vi "Teleop.vi"(10 "Match Info":T1={"Autonomous Elapsed Seconds"=0.0, "TeleOp Elapsed Seconds"=0.0, "Disabled Elapsed Seconds"=0.0, "Visited Autonomous"=FALSE, "Visited TeleOp"=FALSE, "Visited Disabled"=FALSE, "Autonomous Settings"={"Autonomous Style"=enum."Independent", "VI Refnum"=refnum}}, 11 "Call Context":T2) -> ()   [LabVIEW 2019]
doc: "This VI is called for each TeleOp packet received from the DS where the robot is not disabled. It is often used to read from the joysticks and update I/O or to update setpoints for timed control loops. It should complete and return within 20 milliseconds or it may miss DS packets."
uses:
  <vilib>/Rock Robotics/WPI/DriverStation/WPI_DriverStationDerivedRobotMode.ctl
  <vilib>/Rock Robotics/WPI/DriverStation/WPI_DriverStationMatch Info.ctl
  Robot Global Data.vi
  <vilib>/Rock Robotics/Network Tables/NT Write Number.vi
  <vilib>/Rock Robotics/WPI/Utilities/WPI_GetSetVariantRefNum.vi
panel:
  in  "Chassis X SPD":dbl=0.65
  in  "Chassis Y SPD":dbl=0.7
  # "Click here to set max"
  # "Click here to set min"
  # "Click here to set max"
  # "Click here to set min"
  # "Click here to set max"
  # "Click here to set min"
  # "Click here to set max"
  # "Click here to set min"
  # "Click here to set max"
  # "Click here to set min"
  # "Click here to set max"
  # "Click here to set min"
  # "Click here to set max"
  # "Click here to set min"
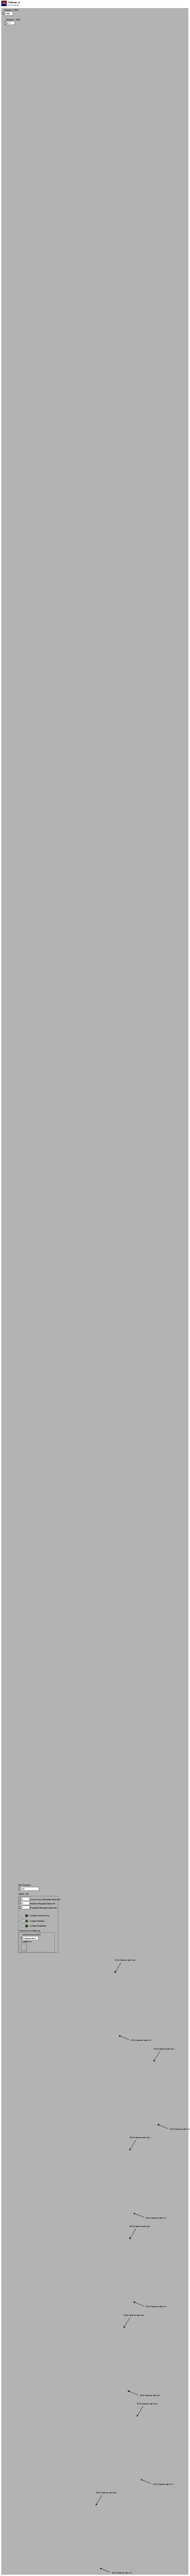
[diagram p1: front panel]
types:
  T1 = typedef "WPI_DriverStationMatch Info.ctl" = cluster{"Autonomous Elapsed Seconds":dbl, "TeleOp Elapsed Seconds":dbl, "Disabled Elapsed Seconds":dbl, "Visited Autonomous":bool, "Visited TeleOp":bool, "Visited Disabled":bool, "Autonomous Settings":cluster{"Autonomous Style":enum16{"Iterative", "Independent"}, "VI Refnum":refnum<vi>}}
  T2 = typedef "WPI_DriverStationDerivedRobotMode.ctl" = enum16{"Init", "Execute", "Stop"}
  T3 = typedef "WPI_MotorControlDeviceRef.ctl" = cluster{"DeviceStatus":errorcluster, "Type":T4, "PWM":cluster{"PWM Channel":T5, "DeadBand":T6}, "CAN":cluster{"Device Number":u8, "SetOutput VI Ref":variant, "GetOutput VI Ref":variant, "Enable VI Ref":variant, "Disable VI Ref":variant, "Data":variant}, "Invert":bool, "DIO PWM":cluster{"PWM \"Enable\" Channel":T5, "DIOChannel":T7, "PWM Rate":dbl}}
  T4 = typedef "WPI_MotorControlType.ctl" = enum16{"PWM", "CAN", "DIO PWM"}
  T5 = typedef "FPGA_DIOPWMChannel.ctl" = enum8{"PWM 0", "PWM 1", "PWM 2", "PWM 3", "PWM 4", "PWM 5", "PWM 6", "PWM 7", "PWM 8", "PWM 9", "PWM MXP 0", "PWM MXP 1", "PWM MXP 2", "PWM MXP 3", "PWM MXP 4", "PWM MXP 5", "PWM MXP 6", "PWM MXP 7", "PWM MXP 8", "PWM MXP 9", "Invalid"}
  T6 = typedef "WPI_PWMDeadband.ctl" = cluster{"Name":string, "maxPositivePwm":i32, "minPositivePwm":i32, "centerPwm":i32, "maxNegativePwm":i32, "minNegativePwm":i32, "angularRange":u16}
  T7 = typedef "FPGA_DIOChannel.ctl" = enum8{"DIO 0", "DIO 1", "DIO 2", "DIO 3", "DIO 4", "DIO 5", "DIO 6", "DIO 7", "DIO 8", "DIO 9", "DIO MXP 0", "DIO MXP 1", "DIO MXP 2", "DIO MXP 3", "DIO MXP 4", "DIO MXP 5", "DIO MXP 6", "DIO MXP 7", "DIO MXP 8", "DIO MXP 9", "DIO MXP 10", "DIO MXP 11", "DIO MXP 12", "DIO MXP 13", "DIO MXP 14", "DIO MXP 15", "SPI Port CS1", "SPI Port CS2", "SPI Port CS3", "SPI Port MISO", "SPI Port MOSI", "Invalid"}
  T8 = typedef "WPI_ServoDeviceRef.ctl" = cluster{"DeviceStatus":errorcluster, "PWM Channel":T5, "DeadBand":T6}
  T9 = typedef "WPI_JoystickDevRef.ctl" = cluster{"Device":T10}
  T10 = typedef "WPI_JoystickDeviceEnum.ctl" = enum16{"USB 0", "USB 1", "USB 2", "USB 3", "USB 4", "USB 5"}
  T11 = typedef "WPI_RobotDriveDevRef.ctl" = cluster{"DevStatus":errorcluster, "Motors[]":T3[], "Square Inputs":bool, "Max Output":dbl}
  T12 = cluster{"JoystickDevRef":T9, "RobotDriveDevRef":T11}
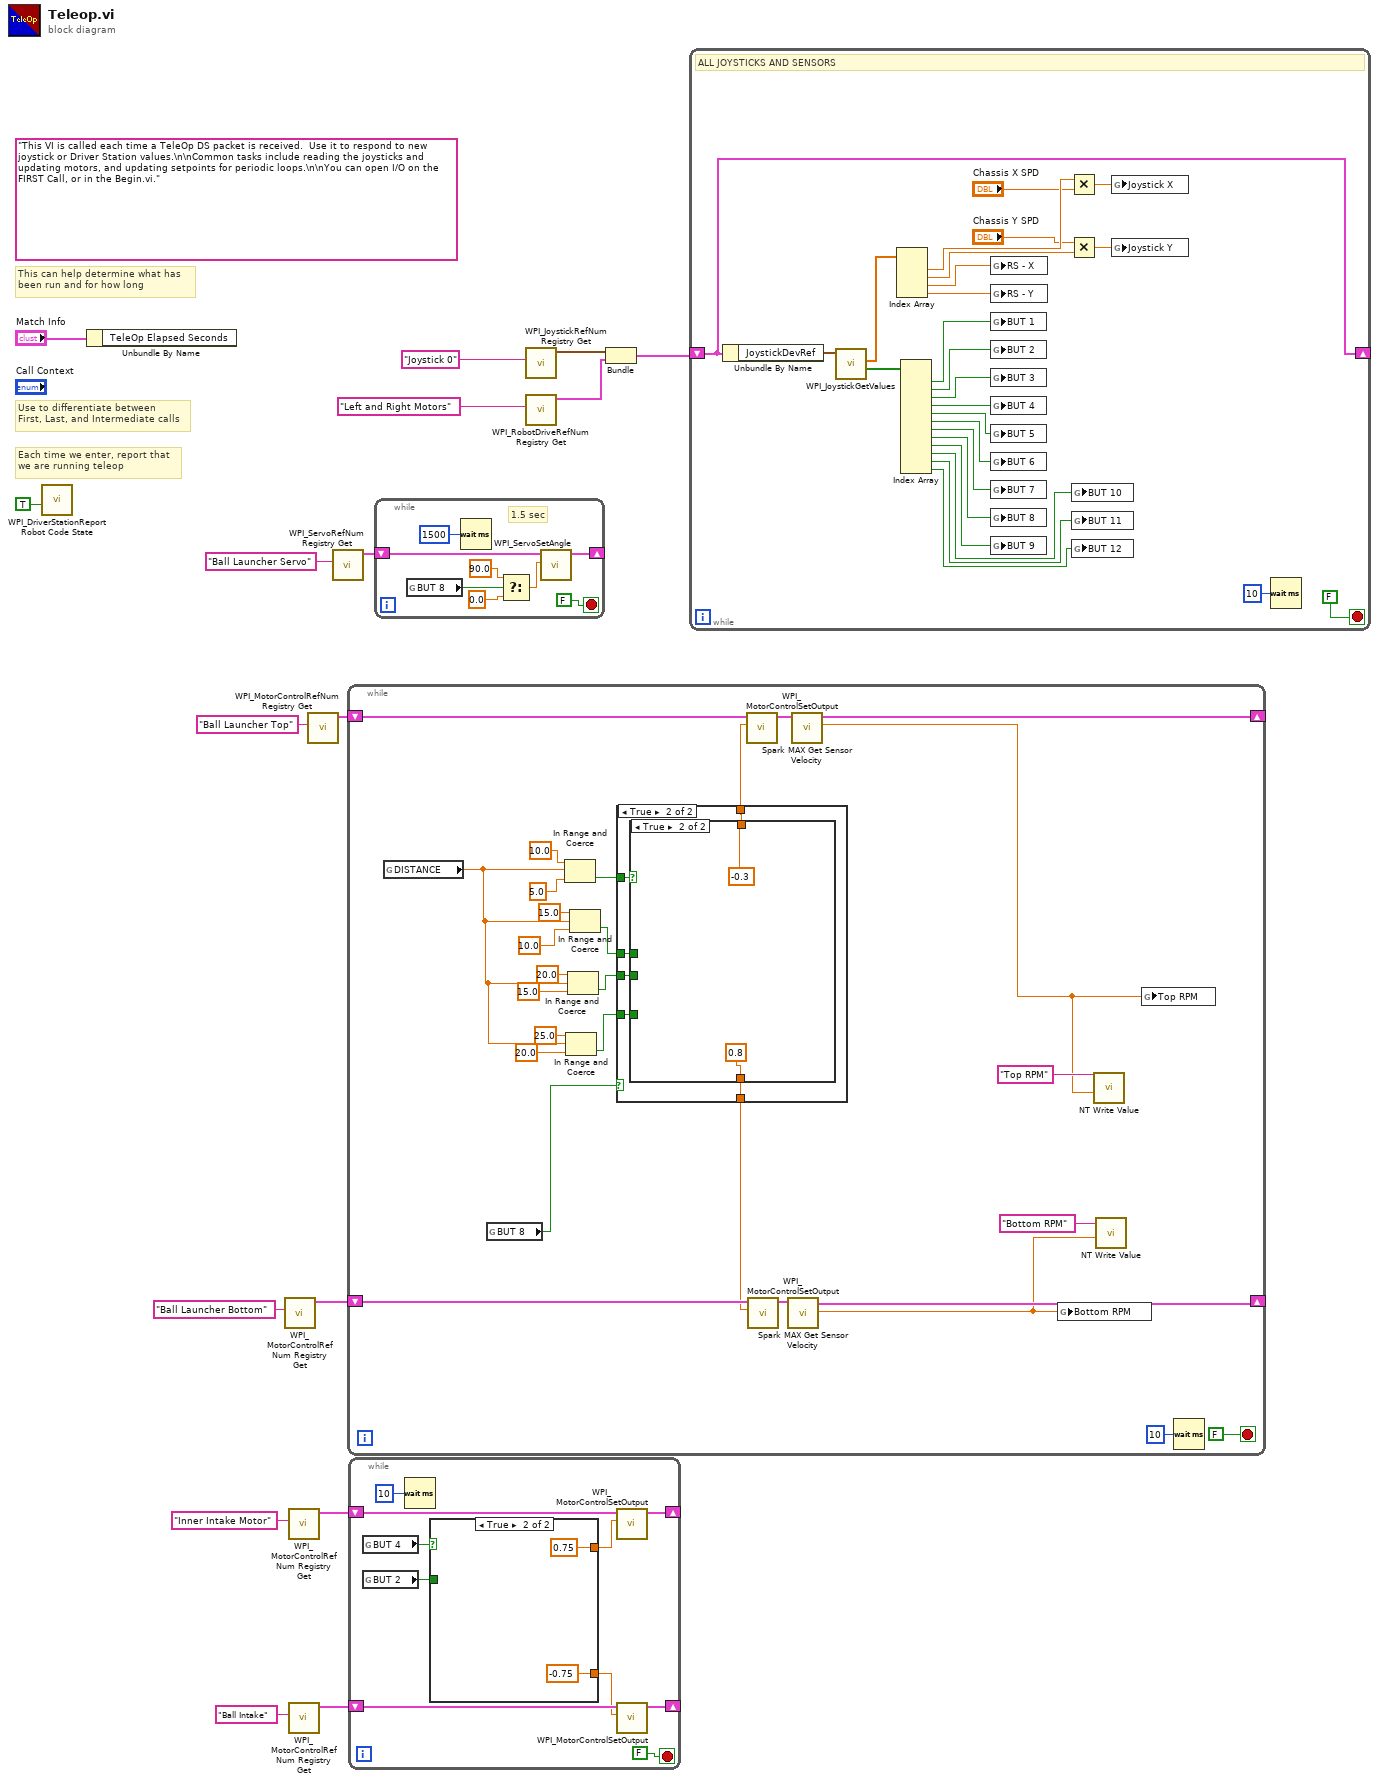
[diagram p0: block diagram]
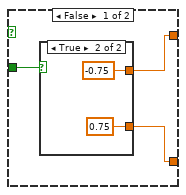
[diagram p2: hidden frame]
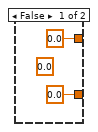
[diagram p3: hidden frame]
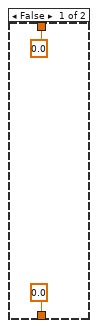
[diagram p4: hidden frame]
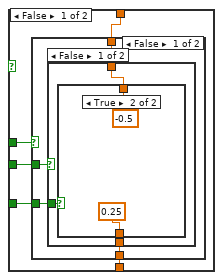
[diagram p5: hidden frame]
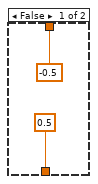
[diagram p6: hidden frame]
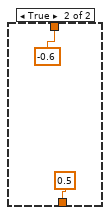
[diagram p7: hidden frame]
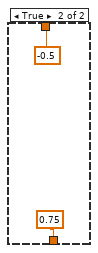
[diagram p8: hidden frame]
diagram:
  (unwired) "This VI is called each time a TeleOp DS packet is received.  Use it to respond to new joystick or Driver Station values.\n\nCommon tasks include reading the joysticks and updating motors, and updating setpoints for periodic loops.\n\nYou can open I/O on the FIRST Call, or in the Begin.vi."
  # "Each time we enter, report that\nwe are running teleop"
  # "Use to differentiate between\nFirst, Last, and Intermediate calls"
  # "This can help determine what has\nbeen run and for how long"
  n1 = call <vilib>:"WPI_DriverStationReport Robot Code State.vi"("TeleOp"=TRUE ("Autonomous")) -> ()  [unwired: 10 in, 1 out]
  n2 = Unbundle By Name("Match Info") -> ()  [unwired: 1 out]
  n3 = call <vilib>:"WPI_MotorControlRefNum Registry Get.vi"("refnum name"="Ball Launcher Bottom") -> ("MotorControlDevRef"=w10:T3)  [unwired: 9 in, 1 out]
  n4 = call <vilib>:"WPI_MotorControlRefNum Registry Get.vi"("refnum name"="Inner Intake Motor") -> ("MotorControlDevRef"=w8:T3)  [unwired: 9 in, 1 out]
  n5 = call <vilib>:"WPI_MotorControlRefNum Registry Get.vi"("refnum name"="Ball Intake") -> ("MotorControlDevRef"=w1:T3)  [unwired: 9 in, 1 out]
  n6 = call <vilib>:"WPI_MotorControlRefNum Registry Get.vi"("refnum name"="Ball Launcher Top") -> ("MotorControlDevRef"=w13:T3)  [unwired: 9 in, 1 out]
  n7 = call <vilib>:"WPI_ServoRefNum Registry Get.vi"("refnum name"="Ball Launcher Servo") -> ("ServoDeviceRef"=w15:T8)  [unwired: 9 in, 1 out]
  n8 = while {
    shift-right: [w33] -> _
    shift-left: w13 -> [w39]
    shift-right: [w41] -> _
    shift-left: w10 -> [w43]
    stop <- FALSE stop-if-true
    n9 = global read "Robot Global Data.vi" "DISTANCE"() -> (w20:dbl)
    n10 = global read "Robot Global Data.vi" "BUT 8"() -> (w19:bool)
    n11 = In Range and Coerce(upper limit=10.0, x=w20, lower limit=5.0) -> (In Range?=w32:bool)  [unwired: 1 out]
    n12 = In Range and Coerce(upper limit=25.0, x=w20, lower limit=20.0) -> (In Range?=w23:bool)  [unwired: 1 out]
    n13 = In Range and Coerce(upper limit=20.0, x=w20, lower limit=15.0) -> (In Range?=w26:bool)  [unwired: 1 out]
    n14 = In Range and Coerce(upper limit=15.0, x=w20, lower limit=10.0) -> (In Range?=w29:bool)  [unwired: 1 out]
    n15 = case shown="True" w19 {
      tunnel: [0.0 ("Output") w53] -> w40
      tunnel: w32 -> [_ w52]
      tunnel: w29 -> [_ w51]
      tunnel: w26 -> [_ w50]
      tunnel: w23 -> [_ w49]
      tunnel: [0.0 ("Output") w48] -> w18
      frame False {
      }
      frame True {
        n16 = case shown="True" w52 {
          tunnel: [w55 -0.3 ("Output")] -> w53
          tunnel: w51 -> [w58 _]
          tunnel: w50 -> [w57 _]
          tunnel: w49 -> [w56 _]
          tunnel: [w54 0.8 ("Output")] -> w48
          frame False {
            n17 = case shown="False" w58 {
              tunnel: w57 -> [w62 _]
              tunnel: w56 -> [w61 _]
              tunnel: [w60 -0.5 ("Output")] -> w55
              tunnel: [w59 0.75 ("Output")] -> w54
              frame False {
                n18 = case shown="False" w62 {
                  tunnel: w61 -> [w65 _]
                  tunnel: [w64 -0.6 ("Output")] -> w60
                  tunnel: [w63 0.5 ("Output")] -> w59
                  frame False {
                    n19 = case shown="True" w65 {
                      tunnel: [-0.5 ("Output") -0.5 ("Output")] -> w64
                      tunnel: [0.5 ("Output") 0.25 ("Output")] -> w63
                      frame False {
                      }
                      frame True {
                      }
                    }
                  }
                  frame True {
                  }
                }
              }
              frame True {
              }
            }
          }
          frame True {
          }
        }
      }
    }
    n20 = call <vilib>:"WPI_MotorControlSetOutput.vi"("Output"=w40, "MotorControlDevRef"=w39) -> ("MotorControlDevRef"=w38:T3)  [unwired: 7 in, 2 out]
    n21 = call <vilib>:"WPI_MotorControlSetOutput.vi"("Output"=w18, "MotorControlDevRef"=w43) -> ("MotorControlDevRef"=w42:T3)  [unwired: 7 in, 2 out]
    n22 = call <vilib>:"Spark MAX Get Sensor Velocity.vi"("MotorControlDevRef in"=w42) -> ("Sensor Velocity"=w34:dbl, "MotorControlDevRef out"=w41:T3)  [unwired: 7 in, 2 out]
    n23 = call <vilib>:"Spark MAX Get Sensor Velocity.vi"("MotorControlDevRef in"=w38) -> ("Sensor Velocity"=w36:dbl, "MotorControlDevRef out"=w33:T3)  [unwired: 7 in, 2 out]
    n24 = global write "Robot Global Data.vi" "Bottom RPM"(w34) -> ()
    n25 = call-poly <vilib>:"NT Write Value.vi"("Numeric"=w36, "Name"="Top RPM") -> ()  [unwired: 9 in, 1 out]
    n26 = call-poly <vilib>:"NT Write Value.vi"("Numeric"=w34, "Name"="Bottom RPM") -> ()  [unwired: 9 in, 1 out]
    n27 = global write "Robot Global Data.vi" "Top RPM"(w36) -> ()
    n28 = Wait (ms)(milliseconds to wait=u32 10) -> ()  [unwired: 1 out]
  }
  n29 = while {
    shift-right: [w84] -> _
    shift-left: w8 -> [w83]
    shift-right: [w78] -> _
    shift-left: w1 -> [w77]
    stop <- FALSE stop-if-true
    n30 = global read "Robot Global Data.vi" "BUT 4"() -> (w81:bool)
    n31 = global read "Robot Global Data.vi" "BUT 2"() -> (w82:bool)
    n32 = Wait (ms)(milliseconds to wait=u32 10) -> ()  [unwired: 1 out]
    n33 = case shown="True" w81 {
      tunnel: [w88 0.75 ("Output")] -> w79
      tunnel: w82 -> [w87 _]
      tunnel: [w86 -0.75 ("Output")] -> w76
      frame False {
        n34 = case shown="True" w87 {
          tunnel: [0.0 ("Output") -0.75 ("Output")] -> w88
          tunnel: [0.0 ("Output") 0.75 ("Output")] -> w86
          frame False {
            (unwired) 0.0 ("Output")
          }
          frame True {
          }
        }
      }
      frame True {
      }
    }
    n35 = call <vilib>:"WPI_MotorControlSetOutput.vi"("Output"=w79, "MotorControlDevRef"=w83) -> ("MotorControlDevRef"=w84:T3)  [unwired: 7 in, 2 out]
    n36 = call <vilib>:"WPI_MotorControlSetOutput.vi"("Output"=w76, "MotorControlDevRef"=w77) -> ("MotorControlDevRef"=w78:T3)  [unwired: 7 in, 2 out]
  }
  n37 = while {
    shift-right: [w98] -> _
    shift-left: w15 -> [w97]
    stop <- FALSE stop-if-true
    # "1.5 sec"
    n38 = global read "Robot Global Data.vi" "BUT 8"() -> (w95:bool)
    n39 = Wait (ms)(milliseconds to wait=u32 1500) -> ()  [unwired: 1 out]
    n40 = Select(t=90.0, s=w95, f=0.0) -> (s? t:f=w96:dbl)
    n41 = call <vilib>:"WPI_ServoSetAngle.vi"("Angle"=w96, "ServoDeviceRef"=w97) -> ("ServoDeviceRef"=w98:T8)  [unwired: 8 in, 1 out]
  }
  n42 = call <vilib>:"WPI_JoystickRefNum Registry Get.vi"("refnum name"="Joystick 0") -> ("JoystickDevRef"=w5:T9)  [unwired: 1 in, 9 out]
  n43 = call <vilib>:"WPI_RobotDriveRefNum Registry Get.vi"("refnum name"="Left and Right Motors") -> ("RobotDriveDevRef"=w4:T11)  [unwired: 1 in, 9 out]
  n44 = Bundle("JoystickDevRef"=w5, "RobotDriveDevRef"=w4) -> (w3:T12)  [unwired: 1 out]
  n45 = while {
    shift-right: [w113] -> _
    shift-left: w3 -> [w113]
    stop <- FALSE stop-if-true
    # "ALL JOYSTICKS AND SENSORS"
    n46 = Unbundle By Name(w113) -> ("JoystickDevRef"=w127:T9)
    n47 = call <vilib>:"WPI_JoystickGetValues.vi"("JoystickDevRef"=w127) -> ("Buttons"=w126:bool[], "Axes"=w112:dbl[])  [unwired: 6 in, 3 out]
    n48 = Index Array(array=w112) -> (element #1=w109:dbl, element #2=w108:dbl, element #3=w105:dbl, element #4=w104:dbl)  [unwired: 4 in]
    n49 = Index Array(array=w126) -> (element #1=w125:bool, element #2=w124:bool, element #3=w123:bool, element #4=w122:bool, element #5=w121:bool, element #6=w120:bool, element #7=w119:bool, element #8=w118:bool, element #9=w117:bool, element #10=w116:bool, element #11=w115:bool, element #12=w114:bool)  [unwired: 12 in]
    n50 = global write "Robot Global Data.vi" "RS - X"(w105) -> ()
    n51 = global write "Robot Global Data.vi" "RS - Y"(w104) -> ()
    n52 = global write "Robot Global Data.vi" "BUT 1"(w125) -> ()
    n53 = global write "Robot Global Data.vi" "BUT 2"(w124) -> ()
    n54 = global write "Robot Global Data.vi" "BUT 3"(w123) -> ()
    n55 = global write "Robot Global Data.vi" "BUT 4"(w122) -> ()
    n56 = global write "Robot Global Data.vi" "BUT 5"(w121) -> ()
    n57 = global write "Robot Global Data.vi" "BUT 6"(w120) -> ()
    n58 = global write "Robot Global Data.vi" "BUT 7"(w119) -> ()
    n59 = global write "Robot Global Data.vi" "BUT 8"(w118) -> ()
    n60 = global write "Robot Global Data.vi" "BUT 9"(w117) -> ()
    n61 = Multiply(x=w109, y="Chassis X SPD") -> (x*y=w111:dbl)
    n62 = Multiply(x="Chassis Y SPD", y=w108) -> (x*y=w110:dbl)
    n63 = global write "Robot Global Data.vi" "BUT 10"(w116) -> ()
    n64 = global write "Robot Global Data.vi" "BUT 11"(w115) -> ()
    n65 = global write "Robot Global Data.vi" "BUT 12"(w114) -> ()
    n66 = global write "Robot Global Data.vi" "Joystick X"(w111) -> ()
    n67 = global write "Robot Global Data.vi" "Joystick Y"(w110) -> ()
    n68 = Wait (ms)(milliseconds to wait=u32 10) -> ()  [unwired: 1 out]
  }
